vi "ManualLauncher.vi"() -> ()   [LabVIEW 2012]
uses:
  LauncherPresets.ctl
  Sally_Dashboard_2014/DBNameEnum.ctl
  Robot Global Data.vi
panel:
  in  "LauncherPresets":T1
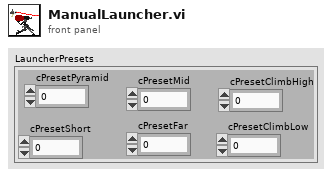
[diagram p1: front panel]
types:
  T1 = typedef "LauncherPresets.ctl" = cluster{"cPresetPyramid":dbl, "cPresetShort":dbl, "cPresetMid":dbl, "cPresetFar":dbl, "cPresetClimbHigh":dbl, "cPresetClimbLow":dbl}
  T2 = typedef "DBNameEnum.ctl" = enum16{"AutoInstructions", "DriveLoopTime", "DriveAlignLSLeft", "DriveAlignLSRight", "Use2DriveAlign", "ClimbLS", "LauncherAngleMatches", "FrameworkVersion", "sLauncherAngle", "LauncherTargetAngle", "sLauncherRPM", "LauncherTargetRPM", "sDriveDistance", "LauncherMotorValue", "PullbackTol", "FireTol", "LauncherRPMTol", "LauncherAngleTol", "InitialWait", "WaitBetweenLaunch", "AnglePresets", "RPMPresets", "UseAngleEncoder", "UseLauncherEncoder", "UseLauncherPID", "QSWaitBeforeFire", "QSWaitBeforeRetract", "AngleForwardValue", "AngleBackwardValue", "UseClusterArray", "BackupAuto", "ReverseDriveIndicate", "HalfSpeedFactor"}
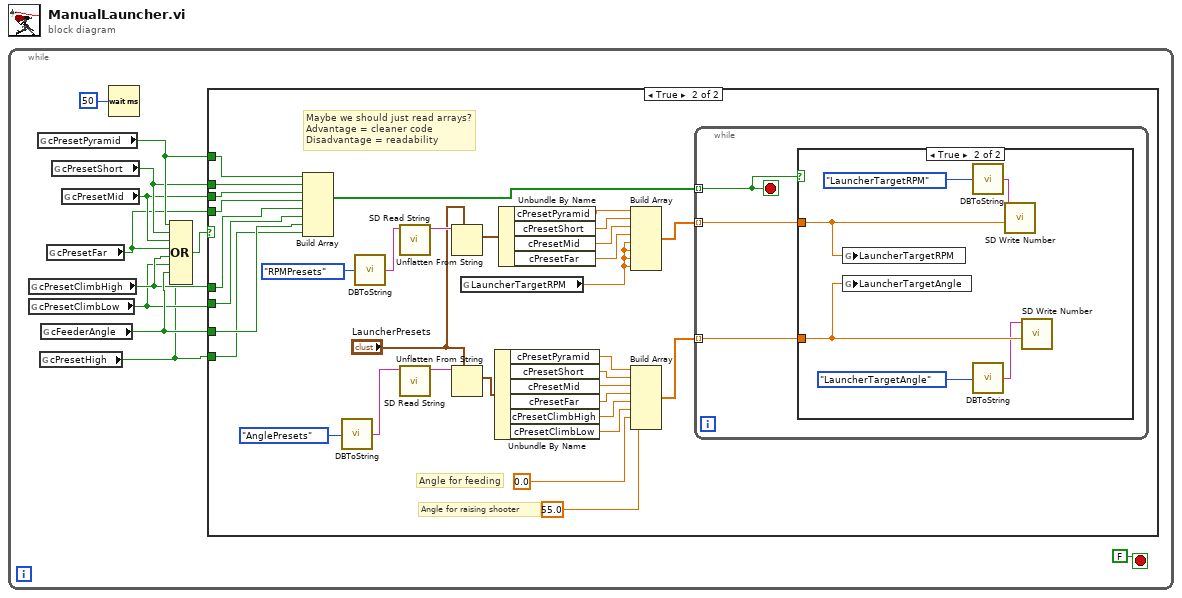
[diagram p0: block diagram]
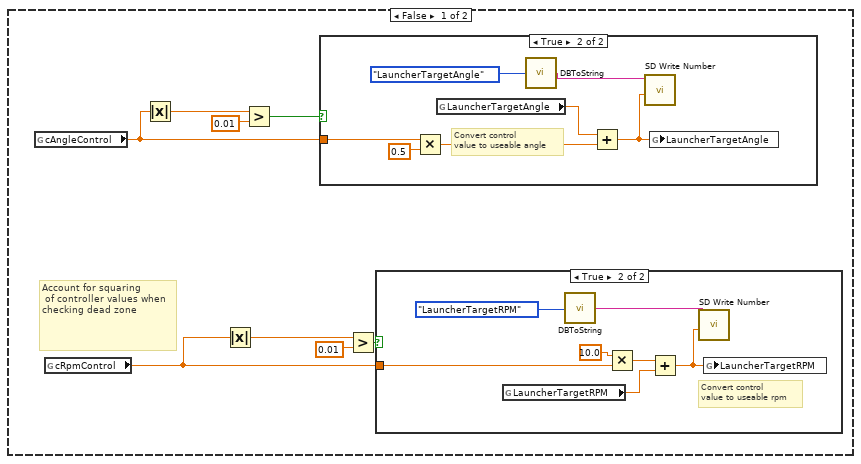
[diagram p2: hidden frame]
diagram:
  n1 = while {
    stop <- FALSE stop-if-true
    n2 = global read "Robot Global Data.vi" "cPresetClimbHigh"() -> (w3:bool)
    n3 = global read "Robot Global Data.vi" "cPresetClimbLow"() -> (w2:bool)
    n4 = global read "Robot Global Data.vi" "cPresetPyramid"() -> (w9:bool)
    n5 = global read "Robot Global Data.vi" "cPresetHigh"() -> (w1:bool)
    n6 = global read "Robot Global Data.vi" "cFeederAngle"() -> (w4:bool)
    n7 = global read "Robot Global Data.vi" "cPresetFar"() -> (w6:bool)
    n8 = global read "Robot Global Data.vi" "cPresetShort"() -> (w8:bool)
    n9 = global read "Robot Global Data.vi" "cPresetMid"() -> (w7:bool)
    n10 = Wait (ms)(milliseconds to wait=u32 50) -> ()  [unwired: 1 out]
    n11 = Compound Arithmetic op=OR(w9, w8, w7, w6, w3, w2, w4, w1) -> (w10:bool)
    n12 = case shown="True" w10 {
      tunnel: w9 -> [_ w66]
      tunnel: w8 -> [_ w65]
      tunnel: w7 -> [_ w64]
      tunnel: w6 -> [_ w63]
      tunnel: w4 -> [_ w37]
      tunnel: w3 -> [_ w39]
      tunnel: w2 -> [_ w38]
      tunnel: w1 -> [_ w36]
      frame False {
        # "Account for squaring\n of controller values when checking dead zone"
        n13 = global read "Robot Global Data.vi" "cAngleControl"() -> (w15:dbl)
        n14 = global read "Robot Global Data.vi" "cRpmControl"() -> (w17:dbl)
        n15 = Absolute Value(x=w15) -> (abs(x)=w16:dbl)
        n16 = Absolute Value(x=w17) -> (abs(x)=w18:dbl)
        n17 = Greater?(x=w16, y=0.01) -> (0:w14:bool)
        n18 = case shown="True" w14 {
          tunnel: w15 -> [_ w26]
          frame False {
          }
          frame True {
            # "Convert control\nvalue to useable angle"
            n19 = Multiply(x=w26, y=0.5) -> (x*y=w23:dbl)
            n20 = global read "Robot Global Data.vi" "LauncherTargetAngle"() -> (w24:dbl)
            n21 = call "DBToString.vi"("Enum"=DBNameEnum."LauncherTargetAngle") -> ("Refname"=w20:string)
            n22 = Add(x=w24, y=w23) -> (x+y=w22:dbl)
            n23 = call <vilib>:"SD Write Number.vi"("Numeric"=w22, "Name"=w20) -> ()  [unwired: 8 in, 2 out]
            n24 = global write "Robot Global Data.vi" "LauncherTargetAngle"(w22) -> ()
          }
        }
        n25 = Greater?(x=w18, y=0.01) -> (0:w13:bool)
        n26 = case shown="True" w13 {
          tunnel: w17 -> [_ w32]
          frame False {
          }
          frame True {
            # "Convert control\nvalue to useable rpm"
            n27 = global read "Robot Global Data.vi" "LauncherTargetRPM"() -> (w31:dbl)
            n28 = call "DBToString.vi"("Enum"=DBNameEnum."LauncherTargetRPM") -> ("Refname"=w27:string)
            n29 = Multiply(x=10.0, y=w32) -> (x*y=w30:dbl)
            n30 = Add(x=w30, y=w31) -> (x+y=w29:dbl)
            n31 = call <vilib>:"SD Write Number.vi"("Numeric"=w29, "Name"=w27) -> ()  [unwired: 8 in, 2 out]
            n32 = global write "Robot Global Data.vi" "LauncherTargetRPM"(w29) -> ()
          }
        }
      }
      frame True {
        # "Angle for raising shooter"
        # "Angle for feeding"
        # "Maybe we should just read arrays?\nAdvantage = cleaner code\nDisadvantage = readability"
        n33 = Build Array(w66, w65, w64, w63, w39, w38, w37, w36) -> (w62:bool[])
        n34 = call "DBToString.vi"("Enum"=DBNameEnum."AnglePresets") -> ("Refname"=w43:string)
        n35 = call "DBToString.vi"("Enum"=DBNameEnum."RPMPresets") -> ("Refname"=w45:string)
        n36 = call <vilib>:"SD Read String.vi"("Name"=w45) -> ("String"=w54:string)  [unwired: 8 in, 2 out]
        n37 = call <vilib>:"SD Read String.vi"("Name"=w43) -> ("String"=w61:string)  [unwired: 8 in, 2 out]
        n38 = Unflatten From String(type="LauncherPresets", binary string=w54) -> (value=w52:T1)  [unwired: 3 in, 2 out]
        n39 = Unflatten From String(type="LauncherPresets", binary string=w61) -> (value=w60:T1)  [unwired: 3 in, 2 out]
        n40 = global read "Robot Global Data.vi" "LauncherTargetRPM"() -> (w35:dbl)
        n41 = Unbundle By Name(w60) -> ("cPresetPyramid"=w59:dbl, "cPresetShort"=w58:dbl, "cPresetMid"=w57:dbl, "cPresetFar"=w56:dbl, "cPresetClimbHigh"=w41:dbl, "cPresetClimbLow"=w40:dbl)
        n42 = Unbundle By Name(w52) -> ("cPresetPyramid"=w51:dbl, "cPresetShort"=w50:dbl, "cPresetMid"=w49:dbl, "cPresetFar"=w48:dbl)
        n43 = Build Array(w51, w50, w49, w48, w35, w35, w35, w35) -> (w47:dbl[])
        n44 = Build Array(w59, w58, w57, w56, w41, w40, 0.0 ("element"), 55.0 ("element")) -> (w55:dbl[])
        n45 = while {
          tunnel: w62 -> [w69] mode=indexing
          tunnel: w55 -> [w68] mode=indexing
          tunnel: w47 -> [w67] mode=indexing
          stop <- w69 stop-if-true
          n46 = case shown="True" w69 {
            tunnel: w68 -> [_ w74]
            tunnel: w67 -> [_ w75]
            frame False {
            }
            frame True {
              n47 = global write "Robot Global Data.vi" "LauncherTargetRPM"(w75) -> ()
              n48 = global write "Robot Global Data.vi" "LauncherTargetAngle"(w74) -> ()
              n49 = call "DBToString.vi"("Enum"=DBNameEnum."LauncherTargetRPM") -> ("Refname"=w72:string)
              n50 = call "DBToString.vi"("Enum"=DBNameEnum."LauncherTargetAngle") -> ("Refname"=w71:string)
              n51 = call <vilib>:"SD Write Number.vi"("Numeric"=w75, "Name"=w72) -> ()  [unwired: 8 in, 2 out]
              n52 = call <vilib>:"SD Write Number.vi"("Numeric"=w74, "Name"=w71) -> ()  [unwired: 8 in, 2 out]
            }
          }
        }
      }
    }
  }
